vi "SOAE-Initialize Acquisition.vi"(0 "Params":T2, 5 "Path":path, 7 "raw data":bool) -> (6 "runtime":T1, 14 "T (ms)":u32, 15 "error out":errorcluster)   [LabVIEW 2020]
uses:
  Typedefs/SOAE-Parameters.ctl
  Typedefs/SOAE-Acq Runtime.ctl
  Utility VIs/Type Defs/Left-Right ring.ctl
  Utility VIs/Math VIs/LinSpace (x0-dx-npts).vi
  Utility VIs/Math VIs/interp1 (1D).vi
panel:
  in  "Header":cluster{"Date":string, "Version":i32}
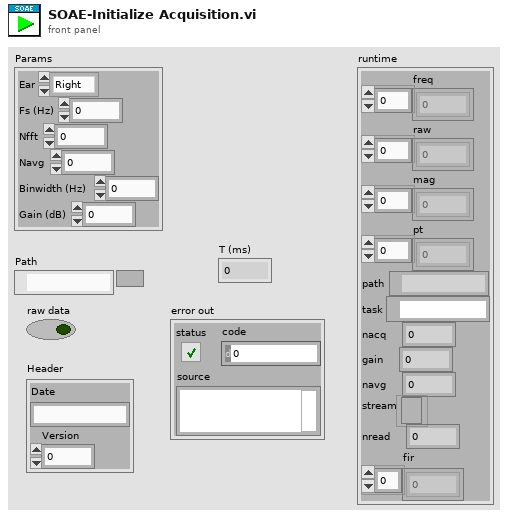
[diagram p1: front panel]
types:
  T1 = typedef "SOAE-Acq Runtime.ctl" = cluster{"freq":dbl[], "raw":dbl[], "mag":dbl[], "pt":dbl[], "path":path, "task":refnum<k21>, "nacq":i32, "gain":dbl, "navg":i32, "stream":refnum<file>, "nread":i32, "fir":dbl[]}
  T2 = typedef "SOAE-Parameters.ctl" = cluster{"Ear":enum16{"Right", "Left"}, "Fs (Hz)":dbl, "Nfft":i32, "Navg":i32, "Binwidth (Hz)":dbl, "Gain (dB)":dbl}
  T3 = typedef "Left-Right ring.ctl" = enum16{"Right", "Left"}
  T4 = enum16{"open", "replace", "create", "open or create", "replace or create", "replace or create with confirmation"}
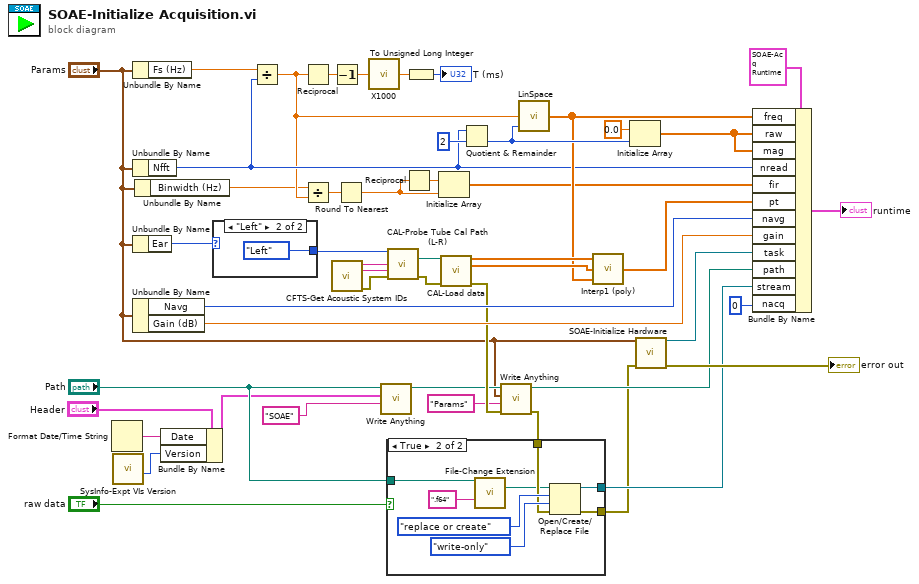
[diagram p0: block diagram]
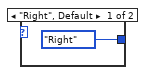
[diagram p2: hidden frame]
diagram:
  n1 = Format Date/Time String() -> (date/time string=w17:string)  [unwired: 3 in]
  n2 = call "SysInfo-Expt VIs Version.vi"() -> ("Expt VIs Version out"=w16:i32)  [unwired: 11 in]
  n3 = Unbundle By Name("Params") -> ("Fs (Hz)"=w47:dbl)
  n4 = Unbundle By Name("Params") -> ("Nfft"=w8:i32)
  n5 = Unbundle By Name("Params") -> ("Ear"=w35:enum16{"Right", "Left"})
  n6 = Unbundle By Name("Params") -> ("Navg"=w29:i32, "Gain (dB)"=w28:dbl)
  n7 = Unbundle By Name("Params") -> ("Binwidth (Hz)"=w6:dbl)
  n8 = Bundle By Name(cluster="Header", "Date"=w17, "Version"=w16) -> (w19:cluster{"Date":string, "Version":i32})
  n9 = case shown="\"Left\"" w35 {
    tunnel: [Left-Right_ring."Right" ("Ear") Left-Right_ring."Left" ("Ear")] -> w49
    frame "Right", Default {
    }
    frame "Left" {
    }
  }
  n10 = Divide(x=w47, y=w8) -> (x/y=w7:dbl)
  n11 = Reciprocal(x=w7) -> (1/x=w33:dbl)
  n12 = Divide(x=w6, y=w7) -> (x/y=w4:dbl)
  n13 = Decrement(x=w33) -> (x-1=w30:dbl)
  n14 = call "CFTS-Get Acoustic System IDs.vi"() -> ("error out"=w13:errorcluster, "Left"=w14:string, "Right"=w15:string)  [unwired: 9 in]
  n15 = Round To Nearest(number=w4) -> (nearest integer value=w1:dbl)
  n16 = call "X1000.vi"("X"=w30) -> ("X/1000"=w32:dbl)
  n17 = call "Write Anything.vi"("Section Name (Name of \"Anything\")"="SOAE" ("Section Name (Name of \"Anything\")"), "Anything"=w19, "Path (dialog)"="Path") -> ("Path out"=w20:path)  [unwired: 7 in, 1 out]
  n18 = call "CAL-Probe Tube Cal Path (L-R).vi"("Ear"=w49, "Right"=w15, "Left"=w14, "error in (no error)"=w13) -> ("Probe Tube Cal Path"=w48:path, "error out"=w41:errorcluster)  [unwired: 10 in]
  n19 = Reciprocal(x=w1) -> (1/x=w2:dbl)
  n20 = To Unsigned Long Integer(number=w32) -> (unsigned 32bit integer=→"T (ms)":u32)
  n21 = Initialize Array(w2, w1) -> (w3:dbl[])
  n22 = call "CAL-Load data.vi"("user path"=w48, "error in (no error)"=w41) -> ("Frequency (Hz)"=w11:dbl[], "Mag"=w10:dbl[], "error out"=w27:errorcluster)  [unwired: 6 in, 5 out]
  n23 = Quotient & Remainder(x=w8, y=2) -> (floor(x/y)=w43:i32)  [unwired: 1 out]
  n24 = call "Write Anything.vi"("Error In"=w27, "Section Name (Name of \"Anything\")"="Params" ("Section Name (Name of \"Anything\")"), "Anything"="Params", "Path (dialog)"=w20) -> ("Error Out"=w23:errorcluster, "Path out"=w25:path)  [unwired: 6 in]
  n25 = case shown="True" "raw data" {
    tunnel: "Path" -> [_ w60]
    tunnel: [_ w57] -> w38
    tunnel: [w52 w56] -> w24
    tunnel: w23 -> [w52 w55]
    frame False {
    }
    frame True {
      n26 = call "File-Change Extension.vi"("Path"=w60, "new extension"=".f64" ("string")) -> ("new path"=w53:path)  [unwired: 13 in]
      n27 = Open/Create/Replace File(file path (use dialog)=w53, error in=w55, operation (0:open)=T4."replace or create", access (0:read/write)=enum16{"read/write", "read-only", "write-only"}."write-only") -> (refnum out=w57:refnum<file>, error out=w56:errorcluster)  [unwired: 2 in, 1 out]
    }
  }
  n28 = call-poly "LinSpace.vi"("npts"=w43, "dx"=w7) -> ("Array"=w9:dbl[])  [unwired: 2 in, 1 out]
  n29 = call-poly "Interp1 (poly).vi"("X"=w11, "Y"=w10, "U"=w9) -> ("V"=w12:dbl[])  [unwired: 2 in]
  n30 = Initialize Array(0.0 ("element"), w43) -> (w42:dbl[])
  n31 = call "SOAE-Initialize Hardware.vi"("Params"="Params", "error in (no error)"=w24) -> ("task out"=w36:refnum<k21>, "error out"=→"error out":errorcluster)  [unwired: 12 in]
  n32 = Bundle By Name(cluster=T1 {"freq"=[], "raw"=[], "mag"=[], "pt"=[], "path"=path "", "task"="", "nacq"=0, "gain"=0.0, "navg"=0, "stream"=refnum, "nread"=0, "fir"=[]} ("DataAcq"), "freq"=w9, "raw"=w42, "mag"=w42, "nread"=w8, "fir"=w3, "pt"=w12, "navg"=w29, "gain"=w28, "task"=w36, "path"=w25, "stream"=w38, "nacq"=0) -> (→"runtime":T1)
